vi "Get Lowest Target.vi"(10 "Enum":enum16{"Top", "Right", "Bottom", "Left"}(ring)=enum."Bottom", 11 "Target Info":T1(array[cluster])) -> (3 "Cluster":T2)   [LabVIEW 2012]
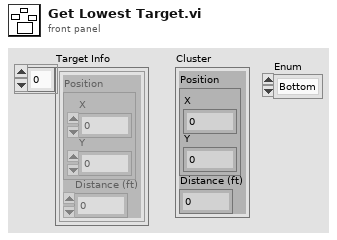
[diagram p1: front panel]
types:
  T1 = cluster{"Position":cluster{"X":dbl, "Y":dbl}, "Distance (ft)":dbl}[]
  T2 = cluster{"Position":cluster{"X":dbl, "Y":dbl}, "Distance (ft)":dbl}
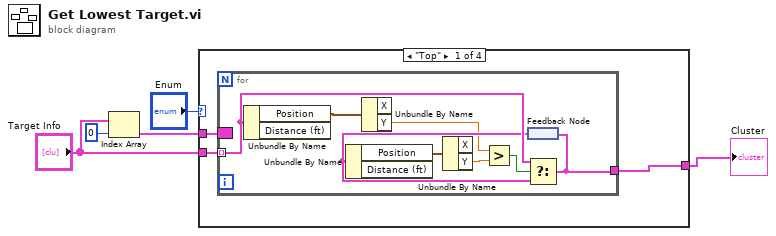
[diagram p0: block diagram]
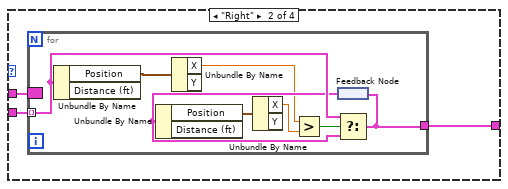
[diagram p2: hidden frame]
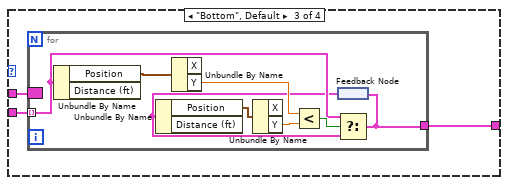
[diagram p3: hidden frame]
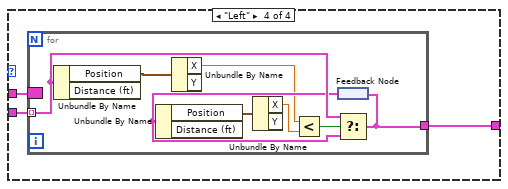
[diagram p4: hidden frame]
diagram:
  n1 = Index Array(array="Target Info", index=0) -> (element=w5:T2)
  n2 = case shown="\"Top\"" "Enum" {
    tunnel: w5 -> [w8 w19 w29 w41]
    tunnel: "Target Info" -> [w7 w18 w30 w40]
    tunnel: [w6 w17 w28 w39] -> w1
    frame "Top" {
      n3 = for {
        tunnel: w7 -> [w14] mode=indexing
        border: w8 -> [_]
        tunnel: [w12] -> w6
        n4 = Unbundle By Name(w14) -> ("Position"=w16:cluster{"X":dbl, "Y":dbl})  [unwired: 1 out]
        n5 = Unbundle By Name(w16) -> ("Y"=w10:dbl)  [unwired: 1 out]
        n6 = feedback #1() -> (w13:T2)
        n7 = Unbundle By Name(w13) -> ("Position"=w15:cluster{"X":dbl, "Y":dbl})  [unwired: 1 out]
        n8 = Unbundle By Name(w15) -> ("Y"=w9:dbl)  [unwired: 1 out]
        n9 = Greater?(x=w10, y=w9) -> (0:w11:bool)
        n10 = Select(t=w14, s=w11, f=w13) -> (s? t:f=w12:T2)
        n11 = feedback-in #1(w12) -> ()
      }
    }
    frame "Right" {
      n12 = for {
        tunnel: w18 -> [w25] mode=indexing
        border: w19 -> [_]
        tunnel: [w23] -> w17
        n13 = Unbundle By Name(w25) -> ("Position"=w27:cluster{"X":dbl, "Y":dbl})  [unwired: 1 out]
        n14 = Unbundle By Name(w27) -> ("X"=w21:dbl)  [unwired: 1 out]
        n15 = feedback #2() -> (w24:T2)
        n16 = Unbundle By Name(w24) -> ("Position"=w26:cluster{"X":dbl, "Y":dbl})  [unwired: 1 out]
        n17 = Unbundle By Name(w26) -> ("X"=w20:dbl)  [unwired: 1 out]
        n18 = Greater?(x=w21, y=w20) -> (0:w22:bool)
        n19 = Select(t=w25, s=w22, f=w24) -> (s? t:f=w23:T2)
        n20 = feedback-in #2(w23) -> ()
      }
    }
    frame "Bottom", Default {
      n21 = for {
        tunnel: w30 -> [w33] mode=indexing
        border: w29 -> [_]
        tunnel: [w31] -> w28
        n22 = Unbundle By Name(w33) -> ("Position"=w38:cluster{"X":dbl, "Y":dbl})  [unwired: 1 out]
        n23 = Unbundle By Name(w38) -> ("Y"=w35:dbl)  [unwired: 1 out]
        n24 = feedback #3() -> (w32:T2)
        n25 = Unbundle By Name(w32) -> ("Position"=w37:cluster{"X":dbl, "Y":dbl})  [unwired: 1 out]
        n26 = Unbundle By Name(w37) -> ("Y"=w34:dbl)  [unwired: 1 out]
        n27 = Less?(x=w35, y=w34) -> (x < y?=w36:bool)
        n28 = Select(t=w33, s=w36, f=w32) -> (s? t:f=w31:T2)
        n29 = feedback-in #3(w31) -> ()
      }
    }
    frame "Left" {
      n30 = for {
        tunnel: w40 -> [w47] mode=indexing
        border: w41 -> [_]
        tunnel: [w45] -> w39
        n31 = Unbundle By Name(w47) -> ("Position"=w49:cluster{"X":dbl, "Y":dbl})  [unwired: 1 out]
        n32 = Unbundle By Name(w49) -> ("X"=w44:dbl)  [unwired: 1 out]
        n33 = feedback #4() -> (w46:T2)
        n34 = Unbundle By Name(w46) -> ("Position"=w48:cluster{"X":dbl, "Y":dbl})  [unwired: 1 out]
        n35 = Unbundle By Name(w48) -> ("X"=w43:dbl)  [unwired: 1 out]
        n36 = Less?(x=w44, y=w43) -> (x < y?=w42:bool)
        n37 = Select(t=w47, s=w42, f=w46) -> (s? t:f=w45:T2)
        n38 = feedback-in #4(w45) -> ()
      }
    }
  }
  "Cluster" <- w1
